vi "WM Ramp up and down.vi"(1 "Ramp Type":enum16{"Linear", "Hanning"}(ring), 2 "Ramp Time":dbl format="%.2f", 3 "Sampling Rate":dbl=1.0 min=0.0 format="%.2f", 4 "Buffer Size":dbl=1.0 min=1.0 format="%.2f") -> (0 "Output":dbl[](array[numeric]) format="%.2f")   [LabVIEW 2012]
uses:
  <vilib>/Analysis/1siggen.llb/Ramp Pattern by Samples.vi
  <vilib>/Analysis/4window.llb/Hanning Window (DBL).vi
  <vilib>/Analysis/NI_AALPro.lvlib
  <vilib>/Analysis/NI_AALBase.lvlib
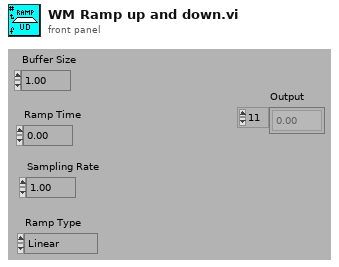
[diagram p1: front panel]
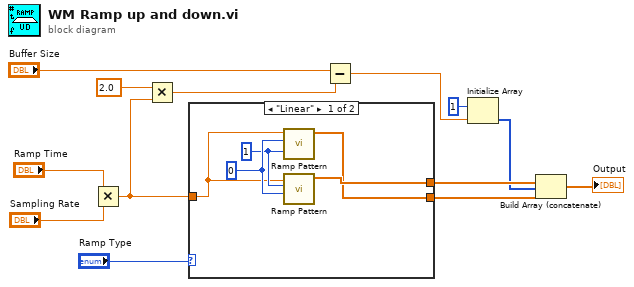
[diagram p0: block diagram]
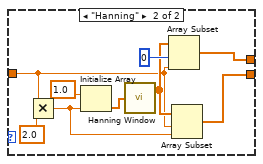
[diagram p2: hidden frame]
diagram:
  n1 = Multiply(x="Ramp Time", y="Sampling Rate") -> (x*y=w2:dbl)
  n2 = Multiply(x=2.0, y=w2) -> (x*y=w12:dbl)
  n3 = case shown="\"Linear\"" "Ramp Type" {
    tunnel: [w17 w23] -> w10
    tunnel: [w16 w19] -> w8
    tunnel: w2 -> [w14 w21]
    frame "Linear" {
      w15 = 1
      w18 = 0
      n4 = call-poly <vilib>:"Ramp Pattern.vi"("start"=w15, "end"=w18, "samples"=w14) -> ("Ramp Pattern"=w16:dbl[])  [unwired: 7 in, 1 out]
      n5 = call-poly <vilib>:"Ramp Pattern.vi"("start"=w18, "end"=w15, "samples"=w14) -> ("Ramp Pattern"=w17:dbl[])  [unwired: 7 in, 1 out]
    }
    frame "Hanning" {
      n6 = Multiply(x=w21, y=2.0) -> (x*y=w20:dbl)
      n7 = Initialize Array(1.0 ("Element Data"), w20) -> (w25:dbl[])
      n8 = call-poly <vilib>:"Hanning Window.vi"("X"=w25) -> ("Windowed X"=w22:dbl[])  [unwired: 1 out]
      n9 = Array Subset(array=w22, index=0 ("Array Index"), length=w21) -> (w23:dbl[])
      n10 = Array Subset(array=w22, index=w21, length=w20) -> (w19:dbl[])
    }
  }
  n11 = Subtract(x="Buffer Size", y=w12) -> (x-y=w11:dbl)
  n12 = Initialize Array(1 ("Element Data"), w11) -> (w9:i32[])
  n13 = Build Array (concatenate)(w10, w9, w8) -> (→"Output":dbl[])
